vi "Draw.vi"(8 "error in (no error)":errorcluster, 11 "Concatenated Shape in":refnum<class "Concatenated Shape.lvclass">) -> (0 "error out":errorcluster, 2 "Picture":picture, 3 "Concatenated Shape out":refnum<class "Concatenated Shape.lvclass">)   [LabVIEW 2017, in "Concatenated Shape.lvclass"]
uses:
  Concatenated Shape.lvclass
  C:/Program Files (x86)/National Instruments/LabVIEW 2017/vi.lib/LIEF/Forms/Layered Shape/Layered Shape.lvclass
  C:/Program Files (x86)/National Instruments/LabVIEW 2017/vi.lib/LIEF/Forms/Shape/Shape.lvclass
  Concatenated Shape.lvclass/Concatenated Shape.ctl
  <vilib>/LIEF/Forms/Layered Shape/Layered Shape.lvclass/Layered Shape.ctl
  <vilib>/LIEF/Forms/Layered Shape/Read Overlays.vi
  <vilib>/LIEF/Forms/Layered Shape/Write Overlays.vi
  <vilib>/LIEF/Forms/Shape/Shape.lvclass
  <vilib>/LIEF/Forms/Layered Shape/Layered Shape.lvclass
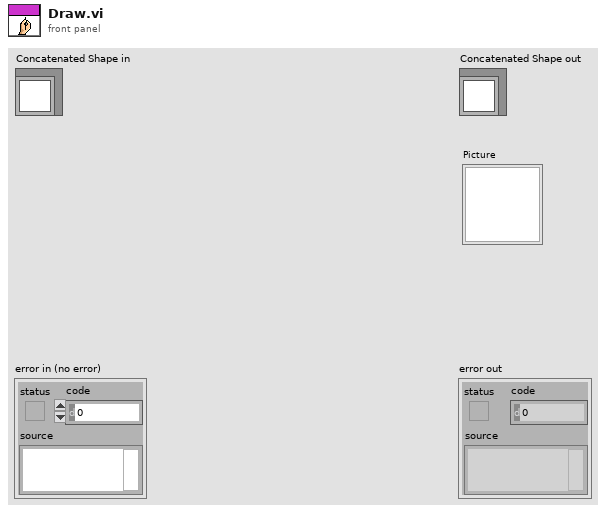
[diagram p1: front panel]
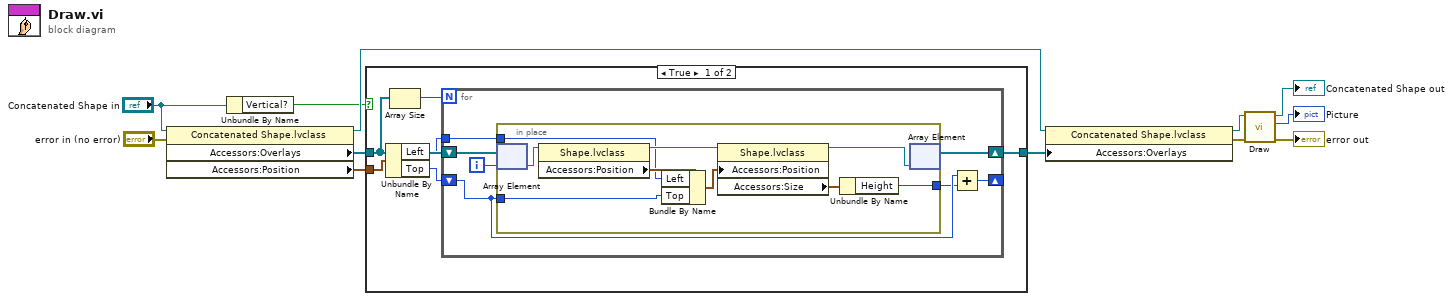
[diagram p0: block diagram]
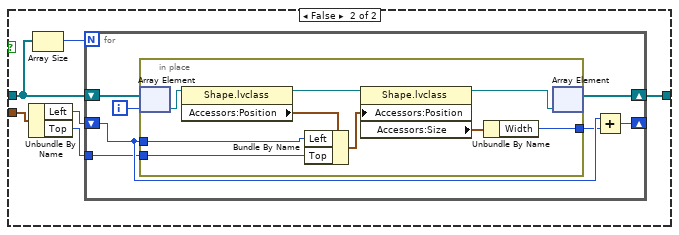
[diagram p2: hidden frame]
diagram:
  n1 = property class="Concatenated Shape.lvclass"(reference="Concatenated Shape in", error in="error in (no error)") -> (reference out=w12:refnum<class "Concatenated Shape.lvclass">, "Accessors:Overlays"=w4:refnum<class "Shape.lvclass">[], "Accessors:Position"=w3:cluster{"Left":i32, "Top":i32})  [unwired: 1 out]
  n2 = Unbundle By Name("Concatenated Shape in") -> ("Vertical?"=w1:bool)
  n3 = case shown="True" w1 {
    tunnel: [w18 w40] -> w11
    tunnel: w4 -> [w17 w39]
    tunnel: w3 -> [w15 w37]
    frame True {
      n4 = Unbundle By Name(w15) -> ("Left"=w13:i32, "Top"=w14:i32)
      n5 = Array Size(array=w17) -> (size(s)=w16:i32)
      n6 = for {
        N: w16 -> [_]
        shift-right: [w21] -> w18
        shift-left: w17 -> [w23]
        shift-right: [w20] -> _
        shift-left: w14 -> [w25]
        tunnel: w13 -> [w19]
        i -> [w22]
        n7 = in-place {
          in-place-border: w25 -> [w30]
          in-place-border: [w27] -> w24
          in-place-border: w19 -> [w26]
          n8 = in-place-array #1(w23, w22) -> (w33:refnum<class "Shape.lvclass">)
          n9 = property class="Shape.lvclass"(reference=w33) -> (reference out=w32:refnum<class "Shape.lvclass">, "Accessors:Position"=w31:cluster{"Left":i32, "Top":i32})  [unwired: 1 in, 1 out]
          n10 = Bundle By Name(cluster=w31, "Left"=w26, "Top"=w30) -> (w29:cluster{"Left":i32, "Top":i32})
          n11 = property class="Shape.lvclass"(reference=w32, "Accessors:Position"=w29) -> (reference out=w34:refnum<class "Shape.lvclass">, "Accessors:Size"=w28:cluster{"Width":i32, "Height":i32})  [unwired: 1 in, 1 out]
          n12 = Unbundle By Name(w28) -> ("Height"=w27:i32)
          n13 = in-place-array #1(w34) -> (w21:refnum<class "Shape.lvclass">[])  [unwired: 1 out]
        }
        n14 = Add(x=w25, y=w24) -> (x+y=w20:i32)
      }
    }
    frame False {
      n15 = Unbundle By Name(w37) -> ("Left"=w36:i32, "Top"=w35:i32)
      n16 = Array Size(array=w39) -> (size(s)=w38:i32)
      n17 = for {
        N: w38 -> [_]
        shift-right: [w43] -> w40
        shift-left: w39 -> [w45]
        shift-right: [w42] -> _
        shift-left: w36 -> [w47]
        tunnel: w35 -> [w41]
        i -> [w44]
        n18 = in-place {
          in-place-border: w47 -> [w52]
          in-place-border: [w49] -> w46
          in-place-border: w41 -> [w48]
          n19 = in-place-array #2(w45, w44) -> (w55:refnum<class "Shape.lvclass">)
          n20 = property class="Shape.lvclass"(reference=w55) -> (reference out=w54:refnum<class "Shape.lvclass">, "Accessors:Position"=w53:cluster{"Left":i32, "Top":i32})  [unwired: 1 in, 1 out]
          n21 = Bundle By Name(cluster=w53, "Left"=w52, "Top"=w48) -> (w51:cluster{"Left":i32, "Top":i32})
          n22 = property class="Shape.lvclass"(reference=w54, "Accessors:Position"=w51) -> (reference out=w56:refnum<class "Shape.lvclass">, "Accessors:Size"=w50:cluster{"Width":i32, "Height":i32})  [unwired: 1 in, 1 out]
          n23 = Unbundle By Name(w50) -> ("Width"=w49:i32)
          n24 = in-place-array #2(w56) -> (w43:refnum<class "Shape.lvclass">[])  [unwired: 1 out]
        }
        n25 = Add(x=w47, y=w46) -> (x+y=w42:i32)
      }
    }
  }
  n26 = property class="Concatenated Shape.lvclass"(reference=w12, "Accessors:Overlays"=w11) -> (reference out=w9:refnum<class "Concatenated Shape.lvclass">, error out=w10:errorcluster)  [unwired: 1 in]
  n27 = call-parent "Draw.vi"("error in (no error)"=w10, "Layered Shape in"=w9) -> ("error out"=→"error out":errorcluster, "Picture"=→"Picture":picture, "Layered Shape out"=→"Concatenated Shape out":refnum<class "Concatenated Shape.lvclass">)  [unwired: 7 in]
